vi "PiezoGlobal.vi"() -> ()   [LabVIEW 2009]
panel:
  out "PiezoGatingTask":refnum<k21>
  out "PiezoWaveformTask":refnum<k21>
  out "PiezoClockingTask":refnum<k21>
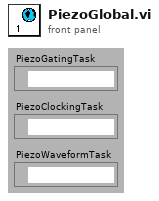
[diagram p1: front panel]
diagram:
